vi "Main -- camera info.vi"() -> ()   [LabVIEW 2013]
uses:
  <vilib>/userdefined/High Color/IMAQdx.ctl
  <vilib>/vision/driver/NI_Vision_Acquisition_Software.lvlib
panel:
  out "video modes":string
  out "attributes":string
  out "all cameras":T1(array[cluster]) {"BusType" format="%x"; "SerialNumberLow" format="%.0x"; "SerialNumberHigh" format="%.0x"}
  in  "webcam":T2="cam0"
  # "LED Matrix demo"
  # "Webcam demo - camera info"
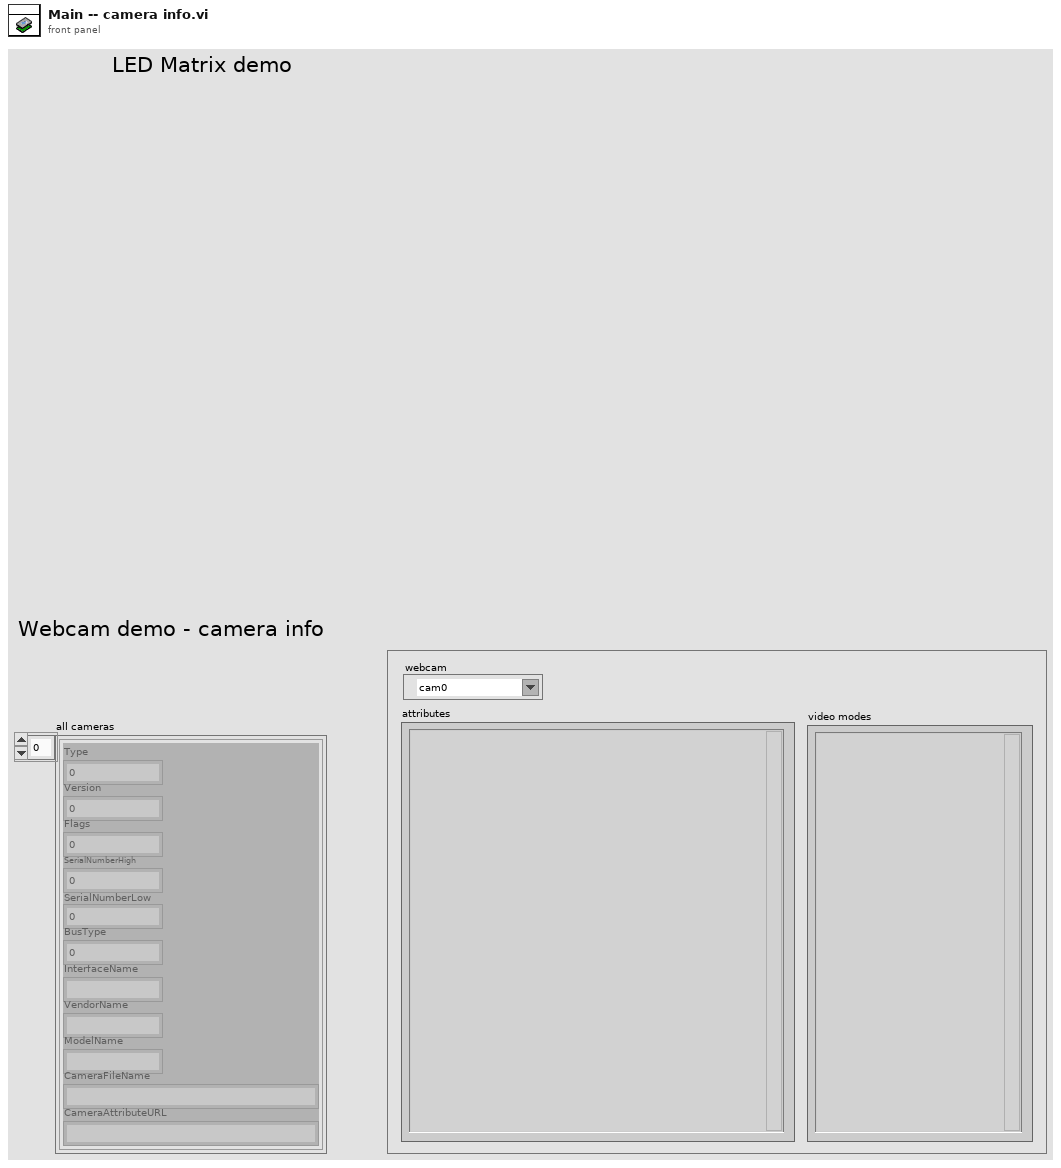
[diagram p1: front panel]
types:
  T1 = cluster{"Type":u32, "Version":u32, "Flags":u32, "SerialNumberHigh":u32, "SerialNumberLow":u32, "BusType":u32, "InterfaceName":string, "VendorName":string, "ModelName":string, "CameraFileName":string, "CameraAttributeURL":string}[]
  T2 = typedef "IMAQdx.ctl" = refnum<k21>
  T3 = typedef "NI_Vision_Acquisition_Software.lvlib/IMAQdx Attribute Type.ctl" = enum32{"U32", "I64", "DBL", "String", "Enum", "Bool", "Command"}
  T4 = cluster{"Attribute Type":T3, "Readable":bool, "Writable":bool, "Attribute Name":string}[]
  T5 = cluster{"Video Mode":u32, "Video Mode Name":string}[]
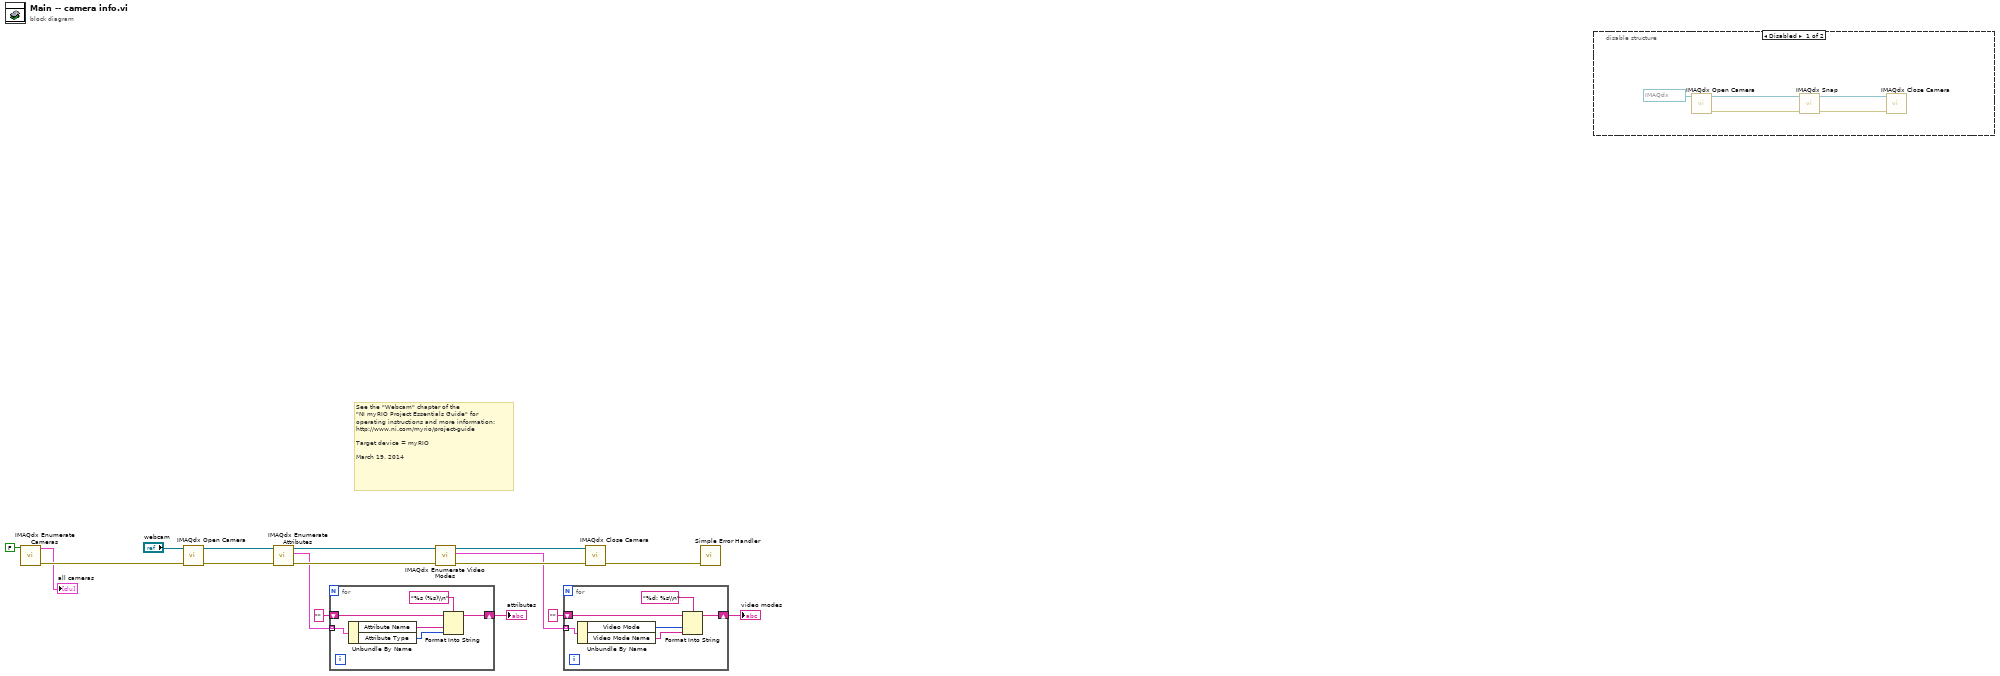
[diagram p0: block diagram]
diagram:
  # "See the \"Webcam\" chapter of the\n\"NI myRIO Project Essentials Guide\" for\noperating instructions and more information: \nhttp://www.ni.com/myrio/project-guide\n\nTarget device = myRIO\n\nMarch 19, 2014"
  n1 = call <vilib>:"IMAQdx Enumerate Cameras.vi"("Connected Only? (Yes)"=FALSE) -> ("error out"=w16:errorcluster, "Camera Information Array"=→"all cameras":T1)  [unwired: 9 in]
  n2 = call <vilib>:"IMAQdx Open Camera.vi"("error in"=w16, "Session In"="webcam") -> ("error out"=w15:errorcluster, "Session Out"=w14:T2)  [unwired: 1 in, 7 out]
  n3 = call <vilib>:"IMAQdx Enumerate Attributes.vi"("error in"=w15, "Session In"=w14) -> ("error out"=w12:errorcluster, "Attribute Information Array"=w6:T4, "Session Out"=w13:T2)  [unwired: 7 in]
  n4 = for {
    tunnel: w6 -> [w23] mode=indexing
    shift-right: [w19] -> w3
    shift-left: "" -> [w18]
    n5 = Unbundle By Name(w23) -> ("Attribute Name"=w21:string, "Attribute Type"=w20:T3)
    n6 = Format Into String(format string="%s (%s)\\n", initial string=w18, w21, w20) -> (resulting string=w19:string)  [unwired: 1 in, 1 out]
  }
  "attributes" <- w3
  n7 = call <vilib>:"IMAQdx Enumerate Video Modes.vi"("error in"=w12, "Session In"=w13) -> ("error out"=w11:errorcluster, "Video Modes"=w5:T5, "Session Out"=w10:T2)  [unwired: 6 in, 1 out]
  n8 = for {
    tunnel: w5 -> [w29] mode=indexing
    shift-right: [w25] -> w4
    shift-left: "" -> [w24]
    n9 = Unbundle By Name(w29) -> ("Video Mode"=w27:u32, "Video Mode Name"=w26:string)
    n10 = Format Into String(format string="%d: %s\\n", initial string=w24, w27, w26) -> (resulting string=w25:string)  [unwired: 1 in, 1 out]
  }
  "video modes" <- w4
  n11 = call <vilib>:"IMAQdx Close Camera.vi"("error in"=w11, "Session In"=w10) -> ("error out"=w9:errorcluster)  [unwired: 9 out]
  n12 = call <vilib>:"Simple Error Handler.vi"("error in (no error)"=w9) -> ()  [unwired: 4 in, 5 out]
  n13 = disable-structure shown="Disabled" {
    frame Disabled {
      n14 = call <vilib>:"IMAQdx Open Camera.vi"("Session In"=T2 "cam0") -> ("error out"=w33:errorcluster, "Session Out"=w32:T2)  [unwired: 9 in]
      n15 = call <vilib>:"IMAQdx Snap.vi"("error in"=w33, "Session In"=w32) -> ("error out"=w31:errorcluster, "Session Out"=w30:T2)  [unwired: 7 in, 1 out]
      n16 = call <vilib>:"IMAQdx Close Camera.vi"("error in"=w31, "Session In"=w30) -> ()  [unwired: 9 in, 1 out]
    }
    frame Enabled {
    }
  }
